vi "MAIN_KD.vi"() -> ()   [LabVIEW 2020]
doc: "Use this template to build a producer/consumer design pattern. Use this template when you need to execute a process, such as data analysis, when a data source, such as a triggered acquisition, produces data at an uneven rate and you need to execute the process when the data becomes available.\n------------------------------------\nAuther: Koji Ohashi\nCopyright (c) 2020 Japan LabVIEW Users Group, Volunteer members.\nThis VI is released under the MIT License.\nhttp://opensource.org/licenses/mit-license.php\n------------------------------------"
uses:
  TESTtypedef UPDATED.ctl
  Angle Target NEW type def.ctl
  states typedef.ctl
  <vilib>/Analysis/baseanly.llb/Mean (DBL).vi
  <vilib>/Instr/_visa.llb/VISA Configure Serial Port (Instr).vi
  <vilib>/Analysis/NI_AALBase.lvlib
  <vilib>/picture/3D Picture Control/NI_3D Picture Control.lvlib
panel:
  in  "Stop":bool
  out "Lab to Arduino":string caption="Participant Name (FirstLast)"
  out "milli timer 3":u32
  out "?":enum32{"Testing", "Init"}(tab)
  out "?":dbl format="%#.3f"
  out "?":u32
  out "?":dbl format="%#.3f"
  out "Tin":dbl format="%#.3f"
  out "?":dbl format="%#.3f"
  out "?":dbl format="%#.3f"
  in  "5":u32(colorbox)
  out "millisecond timer 2":u32
  out "Index (RO)":cluster{"number":dbl, "y1":dbl}(graph)={"number"=2.49, "y1"=0.7722999999999871}
  out "File Name":string caption="Participant Name (FirstLast)"
  in  "File Path":path=path "C:/Users/rsKite/Documents/FSR DATA/samid"
  in  "Trial":string caption="Participant Name (FirstLast)"
  out "Torque":cluster{"Vout(Torque)":dbl, "Torque":dbl}(graph)
  out "Middle (BO)":cluster{"number":dbl, "y1":dbl}(graph)
  in  "Create/Replace":bool
  in  "Folder name":string caption="Participant Name (FirstLast)"
  out "x = y?":bool
  out "Angle":sgl
  out "x*y":dbl
  in  "4":u32(colorbox)
  in  "3":u32(colorbox)
  in  "2":u32(colorbox)
  in  "1":u32(colorbox)
  in  "Stop Test":bool
  in  "Start Test":bool
  out "millisecond timer":u32
  in  "Timer [ms]":u32=5000
  out "On Time [ms]":u32
  in  "Device Angle":enum16{"0", "22.5", "45", "67.5", "90"}(ring)
  in  "Knob Dia":enum16{"2 in", "3 in", "4 in"}(ring)
  in  "Angle Target":T1
  in  "Power":enum16{"Low", "Medium", "High"}(ring)
  in  "Direction":enum16{"CW", "CCW"}(ring)
  in  "Test Type":T2
  out "?":string
  in  "VISA":refnum<visa-resource-name>="COM1"
  out "Calibrating":bool
  in  "Calibration":bool
  out "Thumb (M)":cluster{"number":dbl, "y1":dbl}(graph)
  out "Theta":dbl(knob) scale=-90.0..90.0
  out "Tab Control":enum32{"Static", "Dynamic "}(tab)
  out "3D Static":refnum<vi>(3d-picture)
  out "Dynamic":refnum<vi>(3d-picture)
  # "Status"
  # "Hand Grasp Assessment Device with Variable Resistance Control Center"
  # "Control"
  # "Test Setup"
  # "File Control"
  # "Folder/File Information"
  # "Test Control"
  # "Arduino Communication"
  # "DEFAULT PATHS"
  # "Set 3 to any color"
  # "Set 5 to a different color"
  # "Thumb Force"
  # "Test Time (ms)"
  # "Hand Torque"
  # "Theta"
  # "Middle Force"
  # "Index Force"
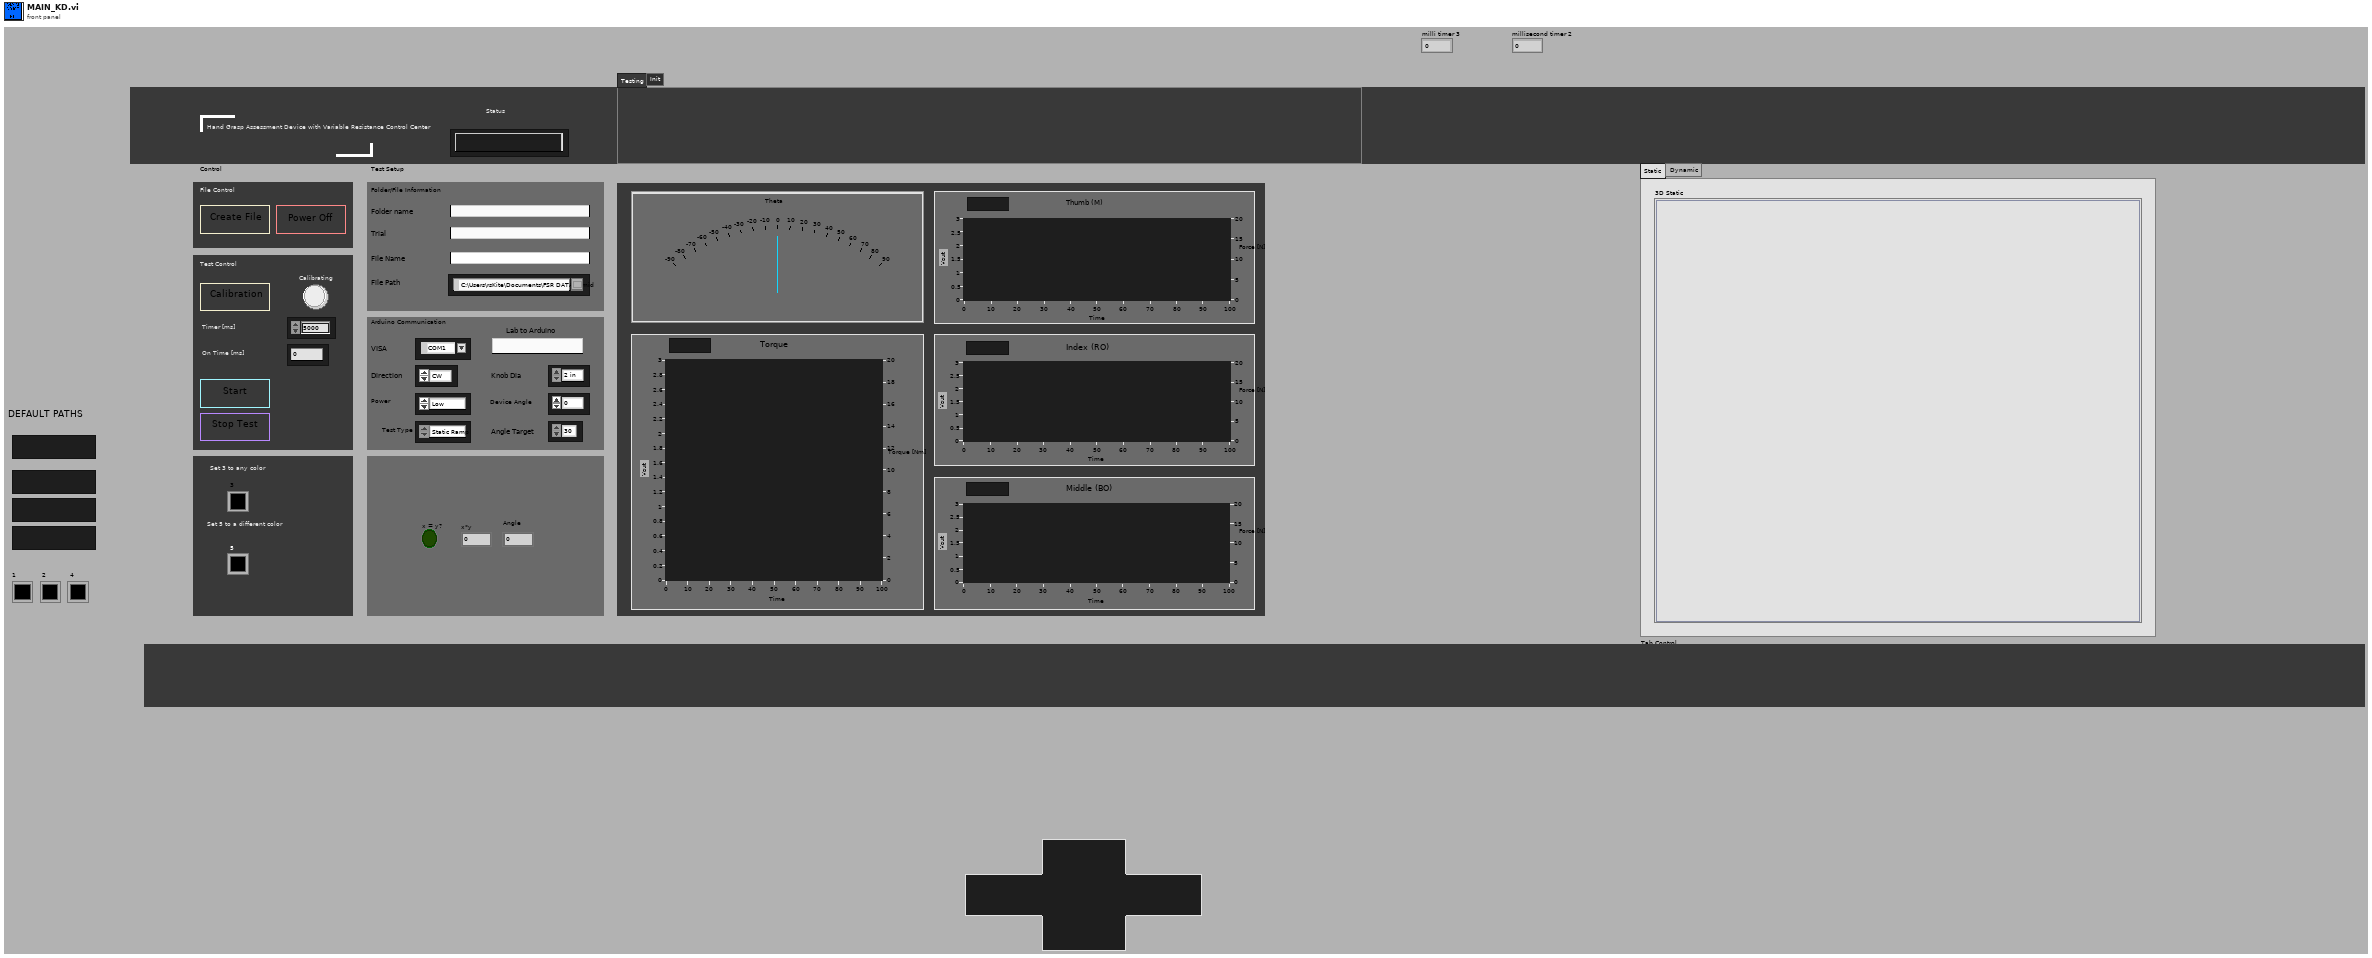
[diagram p1: front panel]
types:
  T1 = typedef "Angle Target NEW type def.ctl" = enum16{"30", "45", "60", "75", "90"}
  T2 = typedef "TESTtypedef UPDATED.ctl" = enum16{"Static Ramp", "Static Sine", "Dynamic"}
  T3 = typedef "states typedef.ctl" = enum16{"Init", "Create/Replace", "Calibration", "Ready?", "Testing", "Write Data", "Restart"}
  T4 = cluster{"String 2":string, "String":string, dbl[], dbl[], dbl[], dbl[], dbl[], dbl[], dbl, "Test Type":T2, "Direction":enum16{"CW", "CCW"}, "Angle Target":T1}
  T5 = cluster{"refnum out":refnum<file>, "error out":errorcluster}
  T6 = cluster{"String 2":string, "String":string, dbl[], dbl[], dbl[], dbl[], dbl[], dbl[], "mean":dbl, "Test Type":T2, "Direction":enum16{"CW", "CCW"}, "Angle Target":T1}
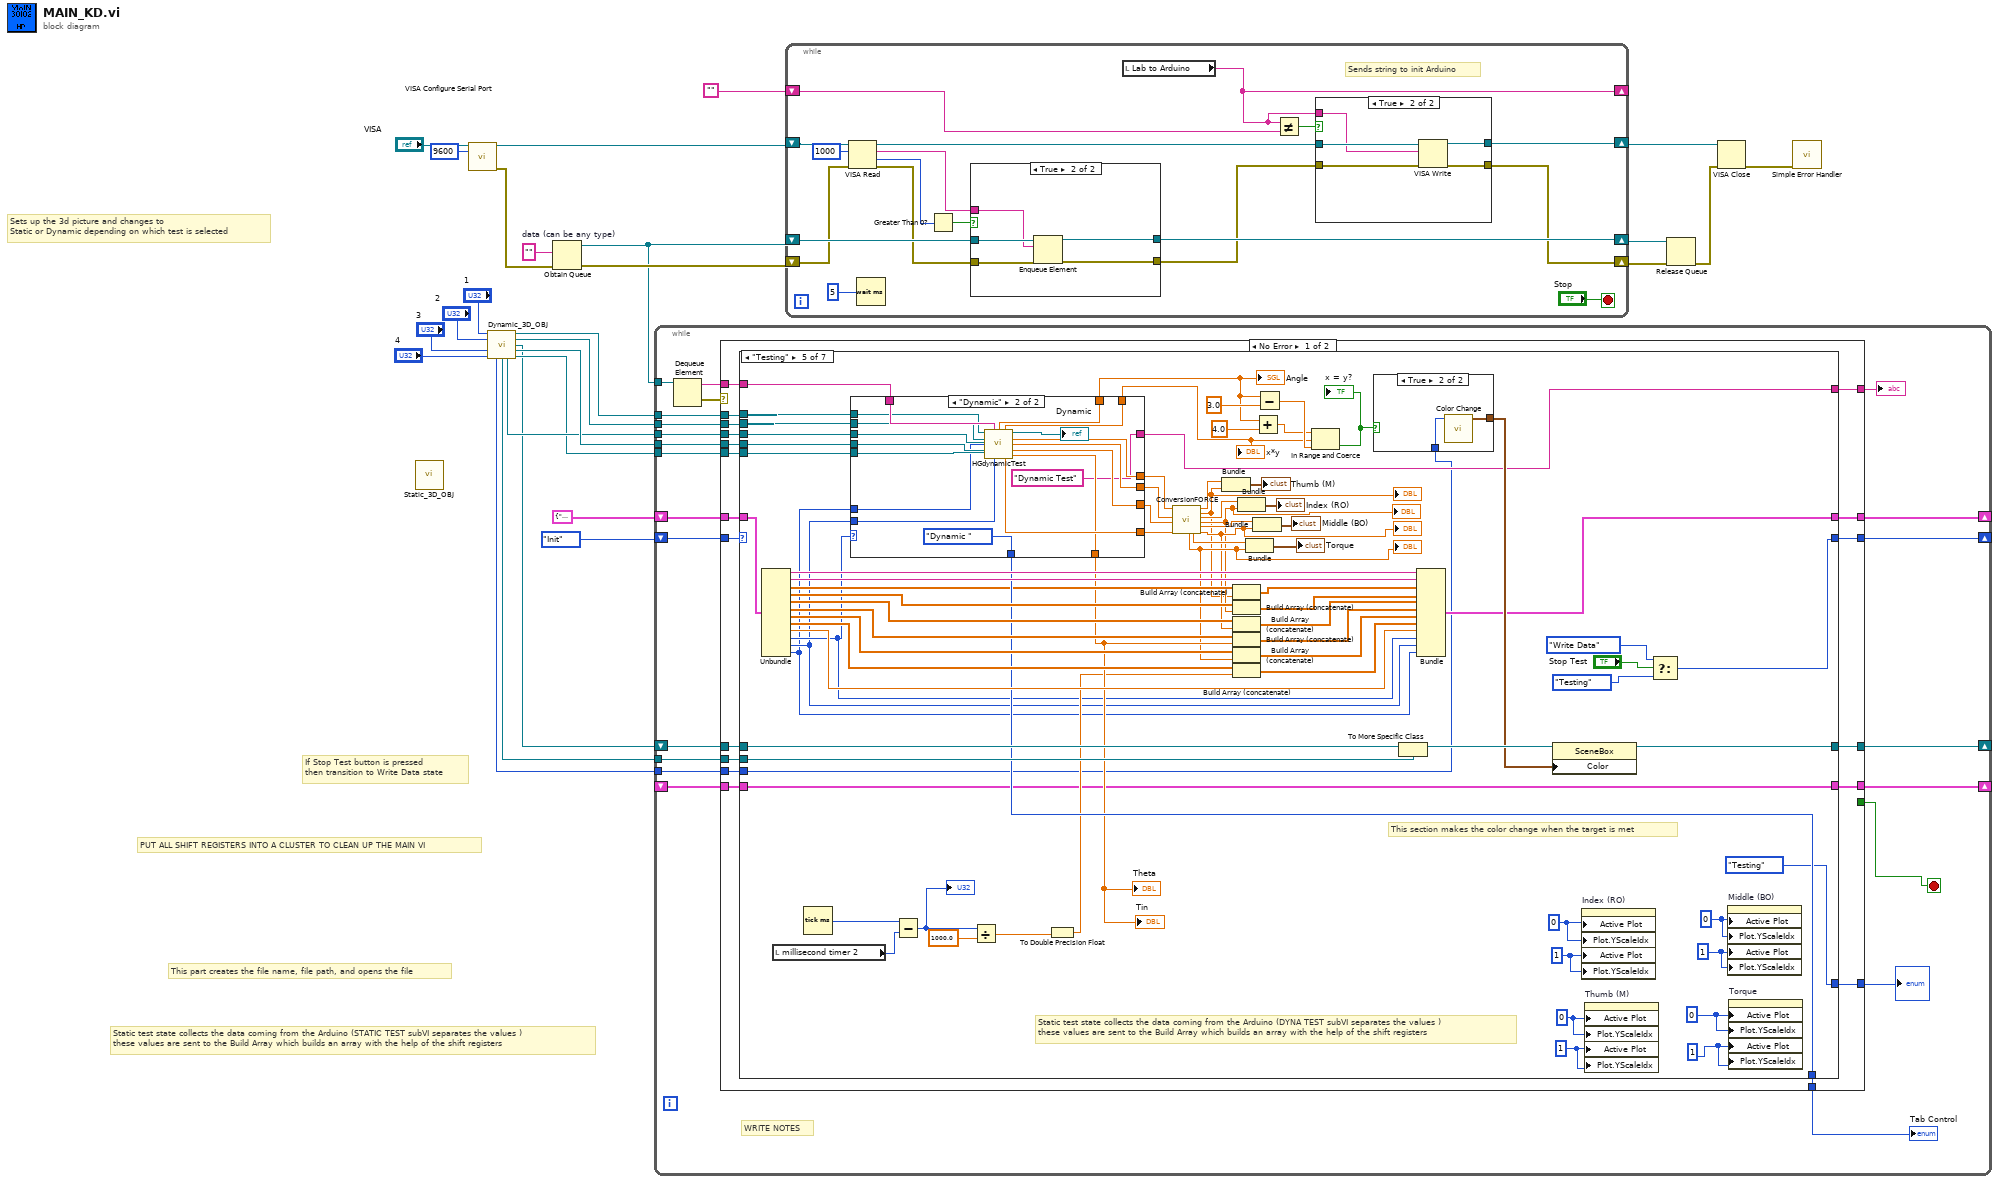
[diagram p0: block diagram]
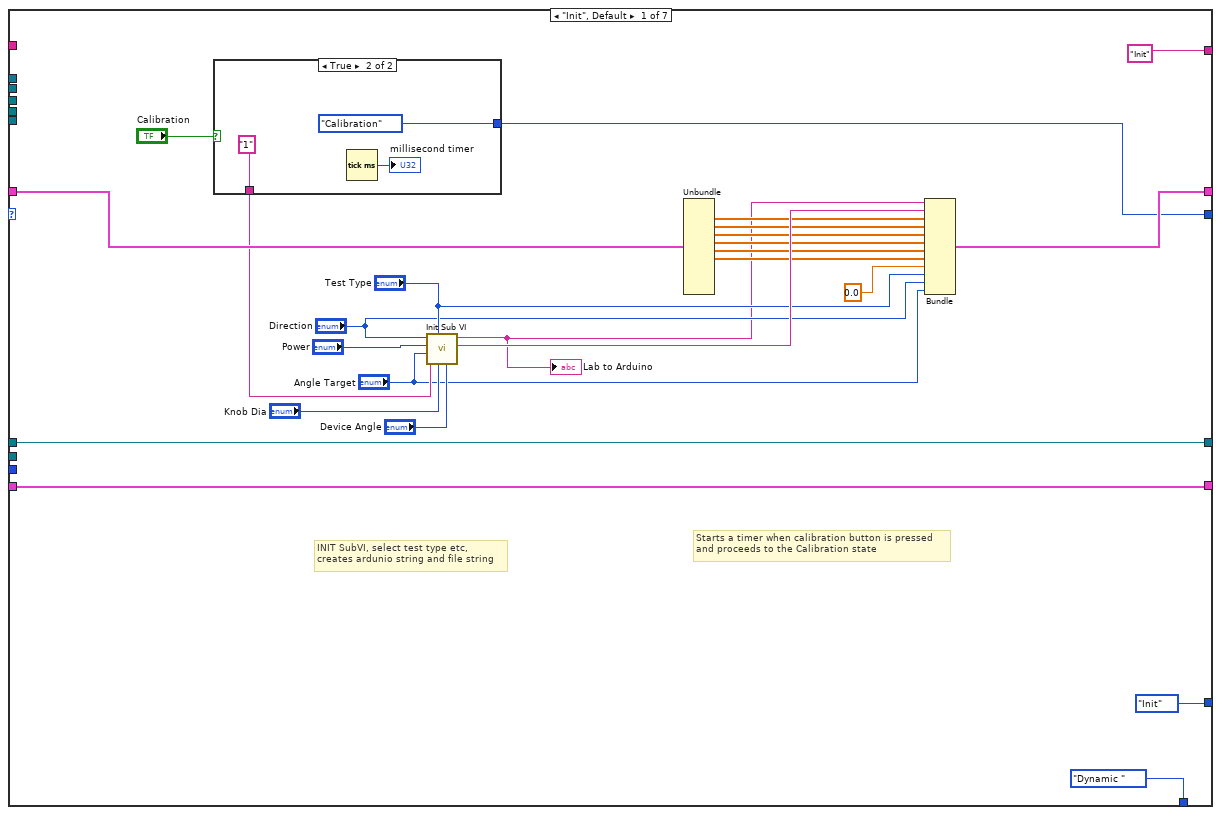
[diagram p2: hidden frame]
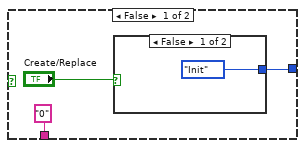
[diagram p3: hidden frame]
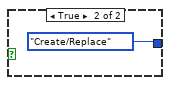
[diagram p4: hidden frame]
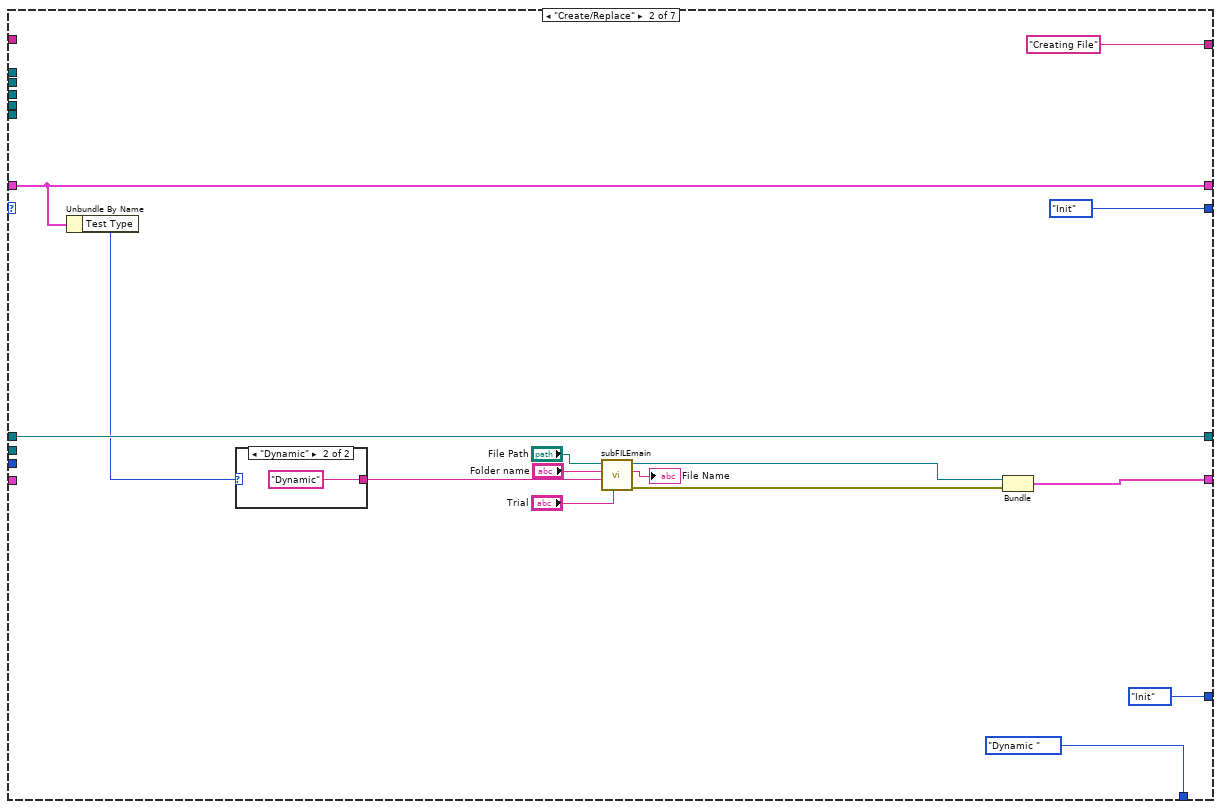
[diagram p5: hidden frame]
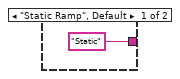
[diagram p6: hidden frame]
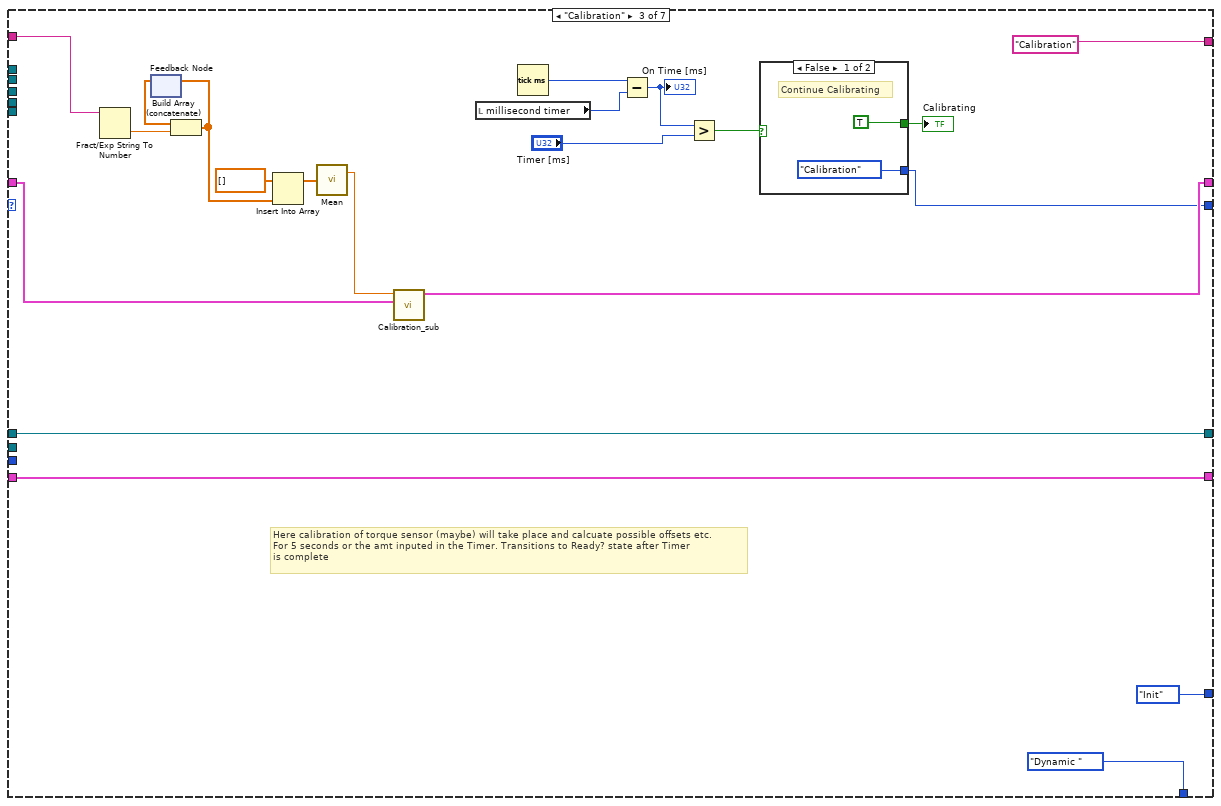
[diagram p7: hidden frame]
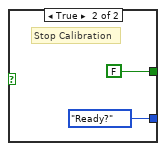
[diagram p8: hidden frame]
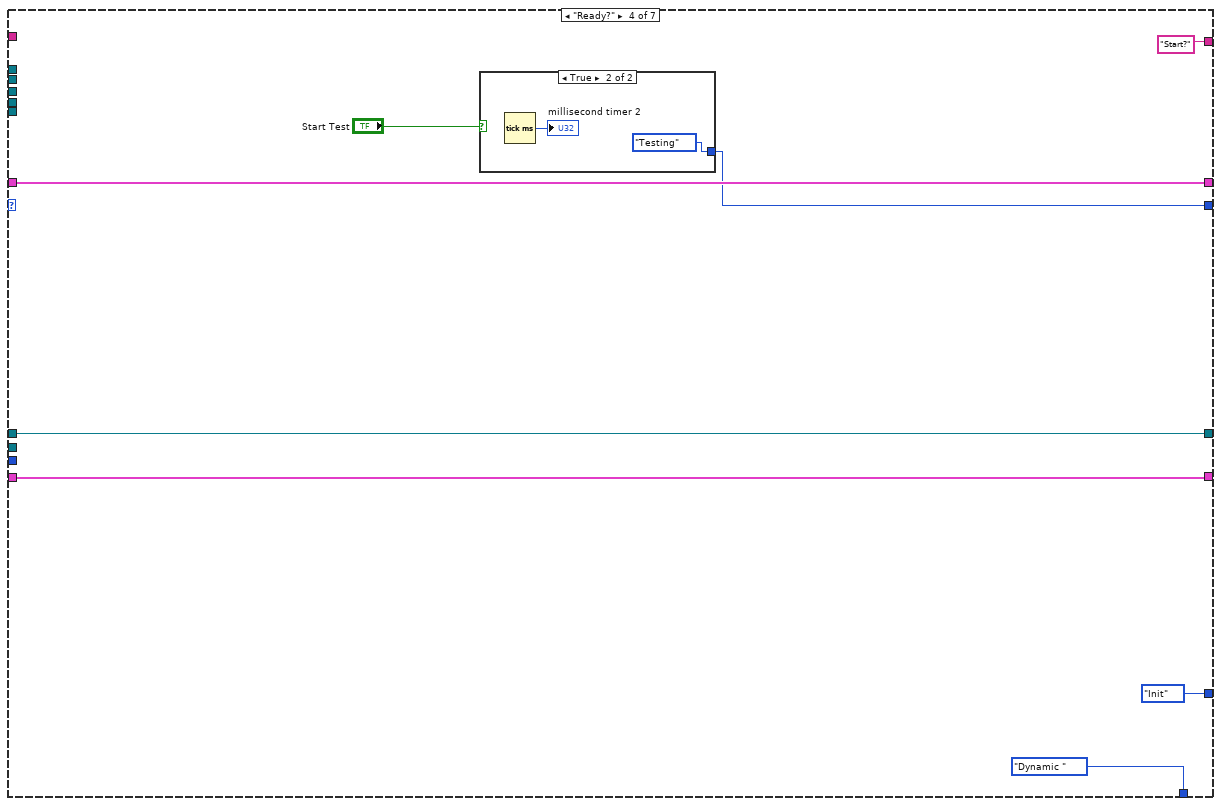
[diagram p9: hidden frame]
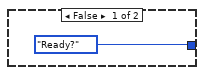
[diagram p10: hidden frame]
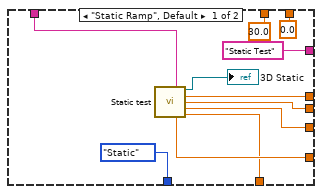
[diagram p11: hidden frame]
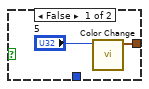
[diagram p12: hidden frame]
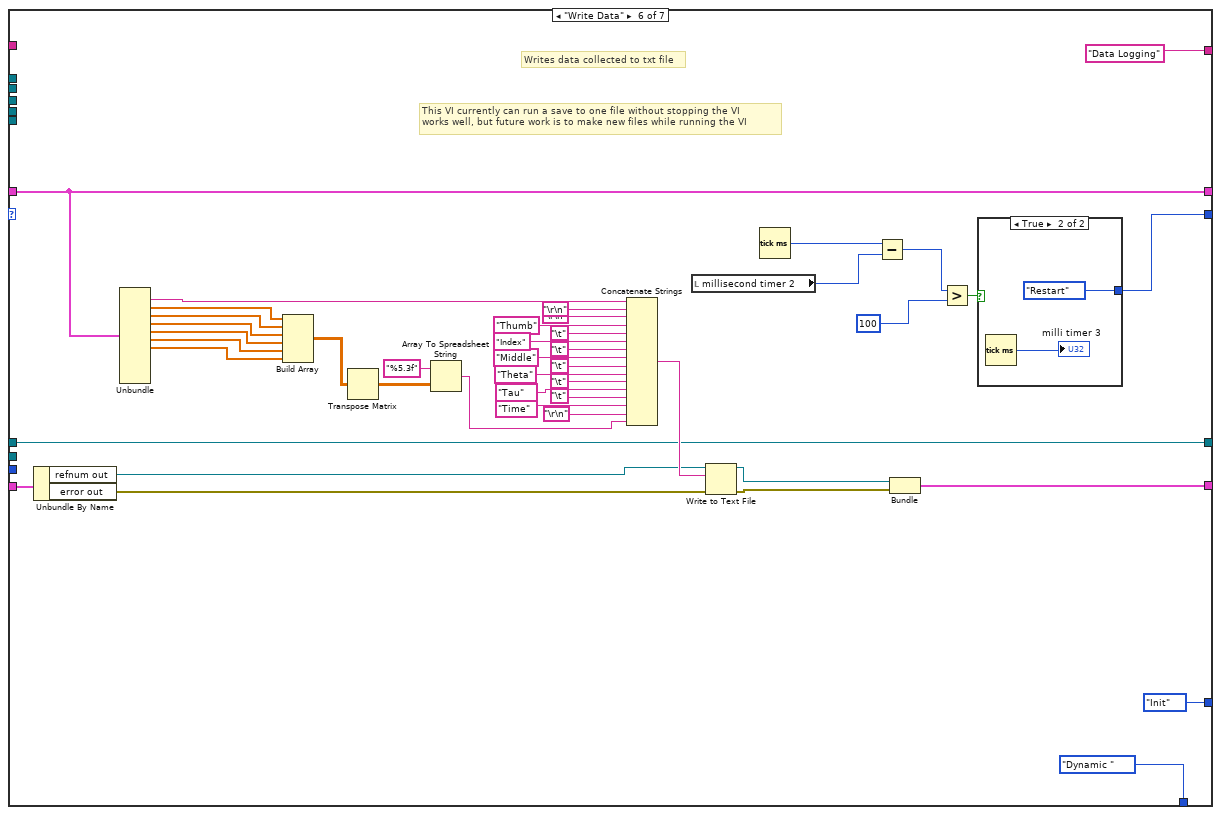
[diagram p13: hidden frame]
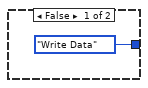
[diagram p14: hidden frame]
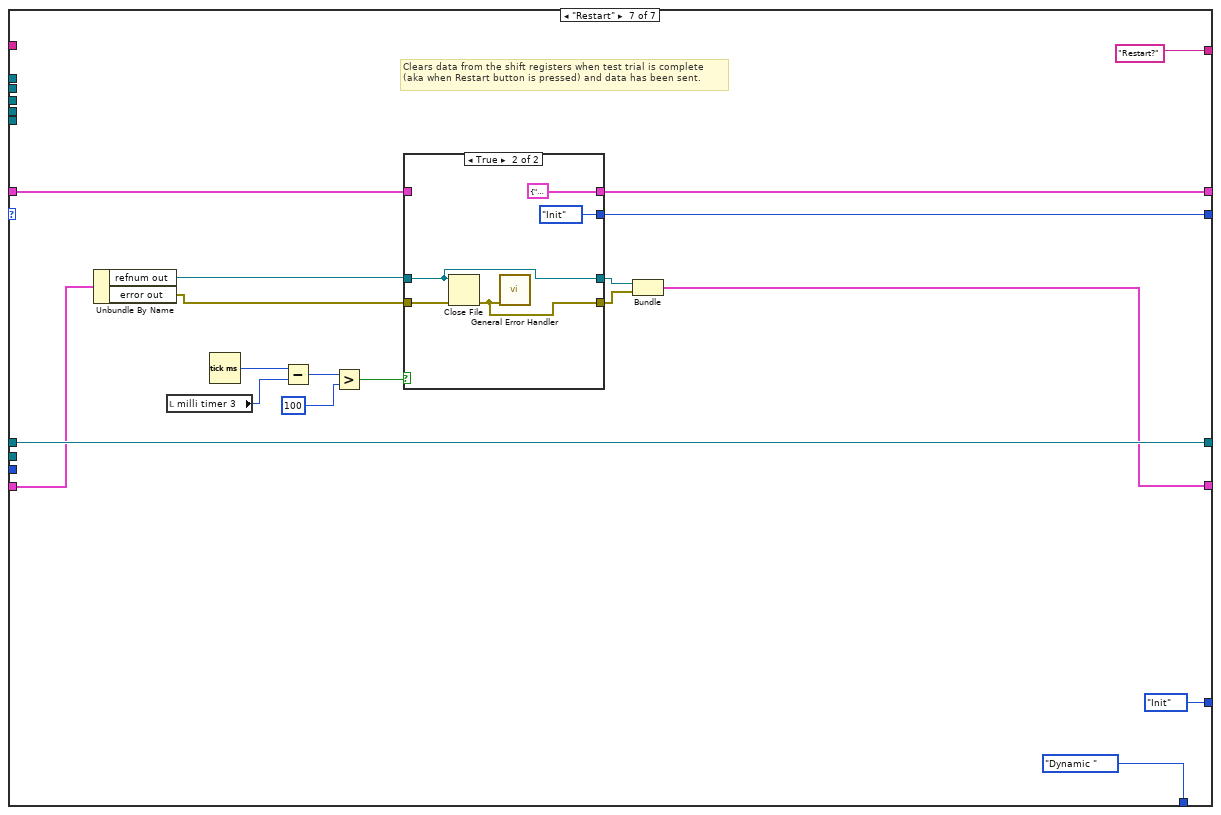
[diagram p15: hidden frame]
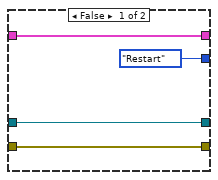
[diagram p16: hidden frame]
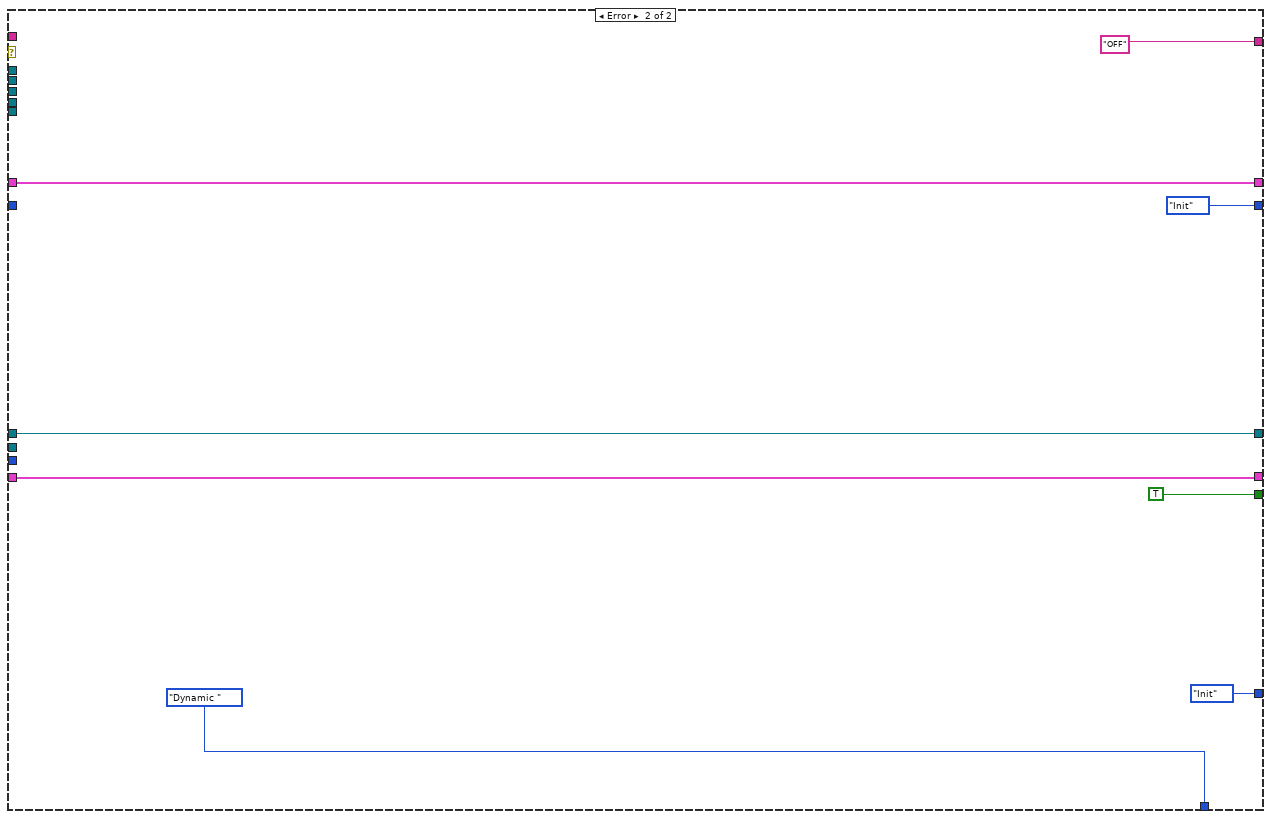
[diagram p17: hidden frame]
diagram:
  w25 = ""  # data (can be any type)
  # "If Stop Test button is pressed \nthen transition to Write Data state"
  # "Static test state collects the data coming from the Arduino (STATIC TEST subVI separates the values ) \nthese values are sent to the Build Array which builds an array with the help of the shift registers"
  # "Sets up the 3d picture and changes to \nStatic or Dynamic depending on which test is selected"
  # "This part creates the file name, file path, and opens the file"
  # "PUT ALL SHIFT REGISTERS INTO A CLUSTER TO CLEAN UP THE MAIN VI"
  n1 = call "Static_3D_OBJ.vi"() -> ()  [unwired: 8 in, 4 out]
  n2 = call-poly "VISA Configure Serial Port"("VISA resource name"="VISA", "baud rate (9600)"=u32 9600) -> ("VISA resource name out"=w26:refnum<visa-resource-name>, "error out"=w23:errorcluster)  [unwired: 8 in, 4 out]
  n3 = call "Dynamic_3D_OBJ.vi"("Color"="1", "Color 2"="2", "Color 3"="3", "Color 4"="4") -> ("SceneObject out"=w13:refnum<vi>, "Child 3"=w12:refnum<vi>, "Drawable"=w3:refnum<vi>, "Child 2"=w11:refnum<vi>, "Color 5"=w1:u32, "New Box Refnum"=w2:refnum<vi>, "Child"=w10:refnum<vi>, "Child 4"=w9:refnum<vi>)  [unwired: 4 in]
  n4 = Obtain Queue(element data type=w25, error in (no error)=w23) -> (queue out=w8:refnum<queue>, error out=w27:errorcluster)  [unwired: 3 in, 1 out]
  n5 = while {
    tunnel: w8 -> [w49]
    shift-right: [w33] -> _
    shift-left: states_typedef."Init" -> [w34]
    shift-right: [w35] -> _
    shift-left: T4 {"String 2"="", "String"="", [], [], [], [], [], [], 0.0, "Test Type"=enum."Dynamic", "Direction"=enum."CW", "Angle Target"=enum."45"} -> [w45]
    tunnel: w13 -> [w44]
    tunnel: w12 -> [w43]
    tunnel: w11 -> [w42]
    tunnel: w10 -> [w41]
    tunnel: w9 -> [w40]
    tunnel: w2 -> [w39]
    shift-right: [w31] -> _
    shift-left: w3 -> [w38]
    shift-right: [w32] -> _
    shift-left: _ -> [w30]
    tunnel: w1 -> [w29]
    stop <- w37 stop-if-true
    # "WRITE NOTES"
    n6 = Dequeue Element(queue=w49) -> (element=w47:string, error out=w48:errorcluster)  [unwired: 2 in, 2 out]
    n7 = case shown="No Error" w48 {
      tunnel: w47 -> [w68 _]
      tunnel: [_ TRUE] -> w37
      tunnel: [w67 "OFF"] -> w46
      tunnel: w45 -> [w66 w343]
      tunnel: w44 -> [w65 _]
      tunnel: w43 -> [w64 _]
      tunnel: w42 -> [w63 _]
      tunnel: w41 -> [w62 _]
      tunnel: w40 -> [w61 _]
      tunnel: w39 -> [w60 _]
      tunnel: w38 -> [w59 w344]
      tunnel: [w53 w344] -> w31
      tunnel: [w57 w343] -> w35
      tunnel: [w58 enum32{"Static", "Dynamic "}."Dynamic " ("Tab Control")] -> w36
      tunnel: w34 -> [w56 _]
      tunnel: [w55 states_typedef."Init"] -> w33
      tunnel: [w54 w340] -> w32
      tunnel: w30 -> [w52 w340]
      tunnel: w29 -> [w51 _]
      tunnel: [w50 enum32{"Testing", "Init"}."Init"] -> w28
      frame No Error {
        n8 = case shown="\"Testing\"" w56 {
          tunnel: w68 -> [_ _ w136 _ w232 _ _]
          tunnel: ["Init" "Creating File" "Calibration" "Start?" w167 "Data Logging" "Restart?"] -> w67
          tunnel: w66 -> [w87 w105 w120 w148 w230 w280 w328]
          tunnel: w65 -> [_ _ _ _ w219 _ _]
          tunnel: w64 -> [_ _ _ _ w218 _ _]
          tunnel: w63 -> [_ _ _ _ w217 _ _]
          tunnel: w62 -> [_ _ _ _ w216 _ _]
          tunnel: w61 -> [_ _ _ _ w192 _ _]
          tunnel: w60 -> [_ _ _ _ w208 _ _]
          tunnel: w59 -> [w86 w106 w126 w150 w207 w294 w327]
          tunnel: [w86 w106 w126 w150 w205 w294 w327] -> w53
          tunnel: [w78 w105 w125 w148 w168 w280 w325] -> w57
          tunnel: [enum32{"Static", "Dynamic "}."Dynamic " ("Tab Control") enum32{"Static", "Dynamic "}."Dynamic " ("Tab Control") enum32{"Static", "Dynamic "}."Dynamic " ("Tab Control") enum32{"Static", "Dynamic "}."Dynamic " ("Tab Control") w178 enum32{"Static", "Dynamic "}."Dynamic " ("Tab Control") enum32{"Static", "Dynamic "}."Dynamic " ("Tab Control")] -> w58
          tunnel: [w75 states_typedef."Init" w122 w146 w164 w278 w318] -> w55
          tunnel: [w73 w107 w121 w145 w163 w267 w319] -> w54
          tunnel: w52 -> [w73 _ w121 w145 w163 w272 w324]
          tunnel: w51 -> [_ _ _ _ w160 _ _]
          tunnel: [enum32{"Testing", "Init"}."Init" enum32{"Testing", "Init"}."Init" enum32{"Testing", "Init"}."Init" enum32{"Testing", "Init"}."Init" enum32{"Testing", "Init"}."Testing" enum32{"Testing", "Init"}."Init" enum32{"Testing", "Init"}."Init"] -> w50
          frame "Init", Default {
            # "INIT SubVI, select test type etc, \ncreates ardunio string and file string"
            # "Starts a timer when calibration button is pressed\nand proceeds to the Calibration state"
            n9 = case shown="True" "Calibration" {
              tunnel: [w95 states_typedef."Calibration"] -> w75
              tunnel: ["0" "1"] -> w74
              frame False {
                n10 = case shown="False" "Create/Replace" {
                  tunnel: [states_typedef."Init" states_typedef."Create/Replace"] -> w95
                  frame False {
                  }
                  frame True {
                  }
                }
              }
              frame True {
                n11 = Tick Count (ms)() -> (millisecond timer value=→"millisecond timer":u32)
              }
            }
            n12 = call "Init Sub VI.vi"("Device Angle"="Device Angle", "Knob Dia"="Knob Dia", "Test Type"="Test Type", "String 3"=w74, "Angle Target"="Angle Target", "Magnitude"="Power", "Direction"="Direction") -> ("String"=w88:string, "String 2"=w69:string)  [unwired: 3 in]
            "Lab to Arduino" <- w69
            n13 = Unbundle(w87) -> (w85:dbl[], w84:dbl[], w83:dbl[], w82:dbl[], w81:dbl[], w80:dbl[])  [unwired: 6 out]
            n14 = Bundle("String 2"=w69, "String"=w88, w85, w84, w83, w82, w81, w80, 0.0, "Test Type"="Test Type", "Direction"="Direction", "Angle Target"="Angle Target") -> (w78:T4)  [unwired: 1 in]
          }
          frame "Create/Replace" {
            n15 = Unbundle By Name(w105) -> ("Test Type"=w104:T2)
            n16 = case shown="\"Dynamic\"" w104 {
              tunnel: ["Static" "Dynamic"] -> w103
              frame "Static Ramp", Default {
              }
              frame "Dynamic" {
              }
            }
            n17 = call "subFILEmain.vi"("Trial"="Trial", "Test"=w103, "Folder name: Participant"="Folder name", "File Folder"="File Path") -> ("error out"=w108:errorcluster, "File Name"=→"File Name":string, "refnum out"=w109:refnum<file>)  [unwired: 5 in]
            n18 = Bundle("refnum out"=w109, "error out"=w108) -> (w107:T5)  [unwired: 1 in]
          }
          frame "Calibration" {
            # "Here calibration of torque sensor (maybe) will take place and calcuate possible offsets etc.\nFor 5 seconds or the amt inputed in the Timer. Transitions to Ready? state after Timer \nis complete"
            n19 = Fract/Exp String To Number(string=w136) -> (number=w138:dbl)  [unwired: 3 in, 1 out]
            n20 = feedback #1() -> (w137:dbl[])  [unwired: 1 in]
            n21 = Build Array (concatenate)(w137, w138) -> (w133:dbl[])
            n22 = feedback-in #1(w133) -> ()
            n23 = Insert Into Array(array=dbl[] [], new element=w133) -> (w135:dbl[])  [unwired: 1 in]
            n24 = call-poly <vilib>:"Mean.vi"("X"=w135) -> ("mean"=w124:dbl)  [unwired: 1 out]
            n25 = call "Calibration_sub.vi"("Cluster in"=w120, "mean"=w124) -> ("output cluster"=w125:T6)  [unwired: 9 in]
            n26 = local read "millisecond timer"() -> (w131:u32)
            n27 = Tick Count (ms)() -> (millisecond timer value=w132:u32)
            n28 = Subtract(x=w132, y=w131) -> (x-y=w130:u32)
            "On Time [ms]" <- w130
            n29 = Greater?(x=w130, y="Timer [ms]") -> (0:w127:bool)
            n30 = case shown="False" w127 {
              tunnel: [states_typedef."Calibration" states_typedef."Ready?"] -> w122
              tunnel: [TRUE FALSE] -> w128
              frame False {
                # "Continue Calibrating"
              }
              frame True {
                # "Stop Calibration"
              }
            }
            "Calibrating" <- w128
          }
          frame "Ready?" {
            n31 = case shown="True" "Start Test" {
              tunnel: [states_typedef."Ready?" states_typedef."Testing"] -> w146
              frame False {
              }
              frame True {
                n32 = Tick Count (ms)() -> (millisecond timer value=→"millisecond timer 2":u32)
              }
            }
          }
          frame "Testing" {
            w193 = u32 1 ("Active Plot")
            w194 = u32 0 ("Active Plot")
            w199 = u32 1 ("Active Plot")
            w200 = u32 0 ("Active Plot")
            w201 = u32 1 ("Active Plot")
            w202 = u32 0 ("Active Plot")
            w203 = u32 1 ("Active Plot")
            w204 = u32 0 ("Active Plot")
            # "This section makes the color change when the target is met"
            # "Static test state collects the data coming from the Arduino (DYNA TEST subVI separates the values ) \nthese values are sent to the Build Array which builds an array with the help of the shift registers"
            n33 = Unbundle(w230) -> ("String 2"=w225:string, "String"=w224:string, w177:dbl[], w229:dbl[], w228:dbl[], w227:dbl[], w226:dbl[], w197:dbl[], "mean"=w191:dbl, "Test Type"=w165:T2, "Direction"=w162:enum16{"CW", "CCW"}, "Angle Target"=w161:T1)
            n34 = local read "millisecond timer 2"() -> (w174:u32)
            n35 = Tick Count (ms)() -> (millisecond timer value=w175:u32)
            n36 = case shown="\"Dynamic\"" w165 {
              tunnel: w232 -> [w243 w261]
              tunnel: w219 -> [_ w260]
              tunnel: w218 -> [_ w259]
              tunnel: w217 -> [_ w258]
              tunnel: w216 -> [_ w257]
              tunnel: [sgl 30.0 ("Angle") w256] -> w214
              tunnel: [0.0 ("x*y") w255] -> w210
              tunnel: w192 -> [_ w254]
              tunnel: [w241 w252] -> w182
              tunnel: [w240 w251] -> w181
              tunnel: [w239 w250] -> w180
              tunnel: [w238 w249] -> w179
              tunnel: [enum32{"Static", "Dynamic "}."Static" ("Tab Control") enum32{"Static", "Dynamic "}."Dynamic " ("Tab Control")] -> w178
              tunnel: [w236 w247] -> w176
              tunnel: ["Static Test" "Dynamic Test"] -> w167
              tunnel: w162 -> [_ w245]
              tunnel: w161 -> [_ w244]
              frame "Static Ramp", Default {
                n37 = call "Static test.vi"("data (can be any type)"=w243) -> ("SceneNode out"=→"3D Static":refnum<vi>, "number"=w241:dbl, "number 2"=w240:dbl, "number 3"=w239:dbl, "number 5"=w238:dbl, "number 4"=w236:dbl)  [unwired: 9 in]
              }
              frame "Dynamic" {
                n38 = call "HGdynamicTest.vi"("SceneObject in"=w260, "data (can be any type)"=w261, "Child 3"=w259, "Angle Target"=w244, "Child 2"=w258, "Child"=w257, "Direction"=w245, "Child 4"=w254) -> ("Angle"=w256:sgl, "x*y"=w255:dbl, "SceneNode out"=→"Dynamic":refnum<vi>, "number"=w252:dbl, "number 2"=w251:dbl, "number 3"=w250:dbl, "number 5"=w249:dbl, "number 4"=w247:dbl)
              }
            }
            "Theta" <- w176
            "x*y" <- w210
            "Angle" <- w214
            "Tin" <- w176
            n39 = Subtract(x=w175, y=w174) -> (x-y=w172:u32)
            "?" <- w172
            n40 = Divide(x=w172, y=1000.0) -> (x/y=w173:dbl)
            n41 = To Double Precision Float(number=w173) -> (double precision float=w170:dbl)
            n42 = call "ConversionFORCE.vi"("number"=w182, "number 2"=w181, "number 3"=w180, "number 4"=w179) -> ("Torque"=w159:dbl, "Vout(Torque)"=w184:dbl, "Vout(M)"=w187:dbl, "Force(M)"=w156:dbl, "Vout(RO)"=w186:dbl, "Force(RO)"=w157:dbl, "Vout(BO)"=w185:dbl, "Force(BO)"=w158:dbl)  [unwired: 8 in]
            "?" <- w159
            "?" <- w158
            "?" <- w157
            "?" <- w156
            n43 = Bundle("Vout(M)"=w187, "Force(M)"=w156) -> (→"Thumb (M)":cluster{"Vout(M)":dbl, "Force(M)":dbl})  [unwired: 1 in]
            n44 = Build Array (concatenate)(w177, w156) -> (w169:dbl[])
            n45 = Build Array (concatenate)(w229, w157) -> (w223:dbl[])
            n46 = Build Array (concatenate)(w228, w158) -> (w222:dbl[])
            n47 = Build Array (concatenate)(w227, w176) -> (w221:dbl[])
            n48 = Build Array (concatenate)(w226, w159) -> (w220:dbl[])
            n49 = Build Array (concatenate)(w197, w170) -> (w196:dbl[])
            n50 = Bundle("Vout(RO)"=w186, "Force(RO)"=w157) -> (→"Index (RO)":cluster{"Vout(RO)":dbl, "Force(RO)":dbl})  [unwired: 1 in]
            n51 = Bundle("Vout(Torque)"=w184, "Torque"=w159) -> (→"Torque":cluster{"Vout(Torque)":dbl, "Torque":dbl})  [unwired: 1 in]
            n52 = Bundle("Vout(BO)"=w185, "Force(BO)"=w158) -> (→"Middle (BO)":cluster{"Vout(BO)":dbl, "Force(BO)":dbl})  [unwired: 1 in]
            n53 = Add(x=w214, y=sgl 4.0) -> (x+y=w211:sgl)
            n54 = Subtract(x=w214, y=sgl 3.0) -> (x-y=w212:sgl)
            n55 = In Range and Coerce(upper limit=w211, x=w210, lower limit=w212) -> (In Range?=w209:bool)  [unwired: 1 out]
            "x = y?" <- w209
            n56 = case shown="True" w209 {
              tunnel: [w263 w265] -> w195
              tunnel: w160 -> [_ w264]
              frame False {
                n57 = call <vilib>:"Color Change.vi"("Color"="5") -> ("RGBA"=w263:cluster{"R":sgl, "G":sgl, "B":sgl, "A":sgl})  [unwired: 10 in]
              }
              frame True {
                n58 = call <vilib>:"Color Change.vi"("Color"=w264) -> ("RGBA"=w265:cluster{"R":sgl, "G":sgl, "B":sgl, "A":sgl})  [unwired: 10 in]
              }
            }
            n59 = To More Specific Class(target class=w208, reference=w207) -> (specific class reference=w206:refnum<vi>)  [unwired: 1 in, 1 out]
            n60 = Bundle("String 2"=w225, "String"=w224, w169, w223, w222, w221, w220, w196, "mean"=w191, "Test Type"=w165, "Direction"=w162, "Angle Target"=w161) -> (w168:T6)  [unwired: 1 in]
            n61 = property class="SceneBox"(reference=w206, "Color"=w195) -> (reference out=w205:refnum<vi>)  [unwired: 1 in, 1 out]
            n62 = property on="Index (RO)" class="WFChart (strict)"("Active Plot"=w202, "Plot.YScaleIdx"=w202, "Active Plot"=w201, "Plot.YScaleIdx"=w201) -> ()  [unwired: 2 in, 2 out]
            n63 = property on="Thumb (M)" class="WFChart (strict)"("Active Plot"=w204, "Plot.YScaleIdx"=w204, "Active Plot"=w203, "Plot.YScaleIdx"=w203) -> ()  [unwired: 2 in, 2 out]
            n64 = Select(t=states_typedef."Write Data", s="Stop Test", f=states_typedef."Testing") -> (s? t:f=w164:T3)
            n65 = property on="Middle (BO)" class="WFChart (strict)"("Active Plot"=w200, "Plot.YScaleIdx"=w200, "Active Plot"=w199, "Plot.YScaleIdx"=w199) -> ()  [unwired: 2 in, 2 out]
            n66 = property on="Torque" class="WFChart (strict)"("Active Plot"=w194, "Plot.YScaleIdx"=w194, "Active Plot"=w193, "Plot.YScaleIdx"=w193) -> ()  [unwired: 2 in, 2 out]
          }
          frame "Write Data" {
            # "Writes data collected to txt file"
            # "This VI currently can run a save to one file without stopping the VI \nworks well, but future work is to make new files while running the VI"
            n67 = Unbundle By Name(w272) -> ("refnum out"=w271:refnum<file>, "error out"=w270:errorcluster)
            n68 = Unbundle(w280) -> ("String"=w295:string, w287:dbl[], w286:dbl[], w285:dbl[], w284:dbl[], w283:dbl[], w282:dbl[])  [unwired: 5 out]
            n69 = Build Array(w287, w286, w285, w284, w283, w282) -> (w281:dbl[][])
            n70 = Transpose Matrix(1:w281) -> (0:w308:dbl[][])
            n71 = Array To Spreadsheet String(array=w308, 3:"%5.3f" ("format string")) -> (spreadsheet string=w288:string)  [unwired: 1 in]
            n72 = Concatenate Strings(w295, "\r\n", "\r\n", "Thumb", "\t", "Index", "\t", "Middle", "\t", "Theta", "\t", "Tau", "\t", "Time", "\r\n", w288) -> (w297:string)
            n73 = local read "millisecond timer 2"() -> (w276:u32)
            n74 = Write to Text File(file (use dialog)=w271, text=w297, error in=w270) -> (refnum out=w269:refnum<file>, error out=w268:errorcluster)  [unwired: 1 in, 1 out]
            n75 = Tick Count (ms)() -> (millisecond timer value=w277:u32)
            n76 = Subtract(x=w277, y=w276) -> (x-y=w275:u32)
            n77 = Bundle("refnum out"=w269, "error out"=w268) -> (w267:T5)  [unwired: 1 in]
            n78 = Greater?(x=w275, y=u32 100) -> (0:w273:bool)
            n79 = case shown="True" w273 {
              tunnel: [states_typedef."Write Data" states_typedef."Restart"] -> w278
              frame False {
              }
              frame True {
                n80 = Tick Count (ms)() -> (millisecond timer value=→"milli timer 3":u32)
              }
            }
          }
          frame "Restart" {
            # "Clears data from the shift registers when test trial is complete \n(aka when Restart button is pressed) and data has been sent."
            n81 = Unbundle By Name(w324) -> ("refnum out"=w323:refnum<file>, "error out"=w322:errorcluster)
            n82 = local read "milli timer 3"() -> (w316:u32)
            n83 = Tick Count (ms)() -> (millisecond timer value=w314:u32)
            n84 = Subtract(x=w314, y=w316) -> (x-y=w315:u32)
            n85 = Greater?(x=w315, y=u32 100) -> (0:w312:bool)
            n86 = case shown="True" w312 {
              tunnel: [states_typedef."Restart" states_typedef."Init"] -> w318
              tunnel: w328 -> [w330 _]
              tunnel: w323 -> [w332 w336]
              tunnel: w322 -> [w331 w337]
              tunnel: [w332 w336] -> w321
              tunnel: [w331 w335] -> w320
              tunnel: [w330 T4 {"String 2"="", "String"="", [], [], [], [], [], [], 0.0, "Test Type"=enum."Dynamic", "Direction"=enum."CW", "Angle Target"=enum."45"}] -> w325
              frame False {
              }
              frame True {
                n87 = Close File(refnum=w336, error in=w337) -> (error out=w335:errorcluster)  [unwired: 1 out]
                n88 = call <vilib>:"General Error Handler.vi"("error in (no error)"=w335) -> ()  [unwired: 10 in, 5 out]
              }
            }
            n89 = Bundle("refnum out"=w321, "error out"=w320) -> (w319:T5)  [unwired: 1 in]
          }
        }
      }
      frame Error {
      }
    }
    "?" <- w46
    "Tab Control" <- w36
    "?" <- w28
  }
  n90 = while {
    shift-right: [w350] -> w19
    shift-left: w27 -> [w358]
    shift-right: [w363] -> w18
    shift-left: w8 -> [w364]
    shift-right: [w352] -> w17
    shift-left: w26 -> [w356]
    shift-right: [w347] -> _
    shift-left: "" -> [w354]
    stop <- "Stop" stop-if-true
    # "Sends string to init Arduino"
    n91 = VISA Read(VISA resource name=w356, byte count=u32 1000, error in (no error)=w358) -> (VISA resource name out=w353:refnum<visa-resource-name>, read buffer=w359:string, return count=w361:u32, error out=w357:errorcluster)
    n92 = Wait (ms)(milliseconds to wait=u32 5) -> ()  [unwired: 1 out]
    n93 = Greater Than 0?(x=w361) -> (x > 0?=w360:bool)
    n94 = case shown="True" w360 {
      tunnel: w364 -> [w373 w378]
      tunnel: [w373 w377] -> w363
      tunnel: w357 -> [w372 w376]
      tunnel: [w372 w375] -> w351
      tunnel: w359 -> [_ w374]
      frame False {
      }
      frame True {
        n95 = Enqueue Element(queue=w378, element=w374, error in (no error)=w376) -> (queue out=w377:refnum<queue>, error out=w375:errorcluster)  [unwired: 1 in, 1 out]
      }
    }
    n96 = local read "Lab to Arduino"() -> (w347:string)
    n97 = Not Equal?(x=w347, y=w354) -> (x != y?=w349:bool)
    n98 = case shown="True" w349 {
      tunnel: w353 -> [w366 w371]
      tunnel: [w366 w370] -> w352
      tunnel: w351 -> [w365 w369]
      tunnel: [w365 w368] -> w350
      tunnel: w347 -> [_ w367]
      frame False {
      }
      frame True {
        n99 = VISA Write(VISA resource name=w371, write buffer=w367, error in (no error)=w369) -> (VISA resource name out=w370:refnum<visa-resource-name>, error out=w368:errorcluster)  [unwired: 1 out]
      }
    }
  }
  n100 = Release Queue(queue=w18, error in (no error)=w19) -> (error out=w21:errorcluster)  [unwired: 1 in, 2 out]
  n101 = VISA Close(VISA resource name=w17, error in (no error)=w21) -> (error out=w20:errorcluster)
  n102 = call <vilib>:"Simple Error Handler.vi"("error in (no error)"=w20) -> ()  [unwired: 1 in, 8 out]
